vi "CMD_AUTOFOCUS.vi"(6 "Gantry in":refnum<class "Gantry.lvclass">, 8 "error in (no error)":errorcluster, 10 "Arguments":string[](array[string]), 11 "gScript Interpreter in":refnum<class "gScript Interpreter.lvclass">) -> (0 "error out":errorcluster, 3 "gScript Interpreter out":refnum<class "gScript Interpreter.lvclass">, 4 "Gantry out":refnum<class "Gantry.lvclass">)   [LabVIEW 2017, in "gScript Interpreter.lvclass"]
uses:
  gScript Interpreter.lvclass
  Shared Components/Gantry Class/Gantry.lvclass
  Shared Components/Vec3d Class/Vec3d.lvclass
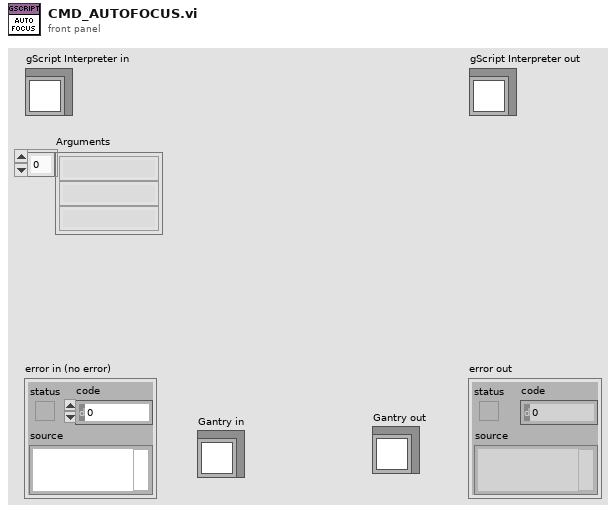
[diagram p1: front panel]
types:
  T1 = typedef "Memory Cell.ctl" = cluster{"type":T2, "x":dbl, "y":dbl, "z":dbl, "w":dbl}
  T2 = typedef "Memory Cell Type Enum.ctl" = enum16{"integer", "float", "vector", "rotation"}
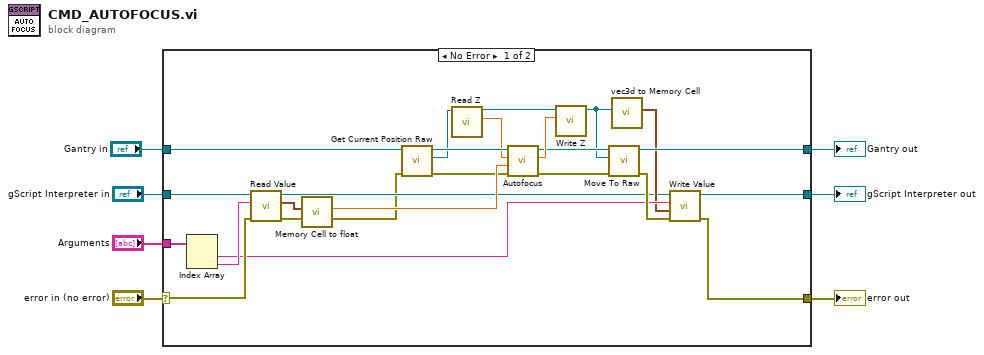
[diagram p0: block diagram]
diagram:
  n1 = case shown="No Error" "error in (no error)" {
    selector: "error in (no error)" -> [w25 w34]
    tunnel: [w27 w34] -> w6
    tunnel: [w29 w33] -> w4
    tunnel: "gScript Interpreter in" -> [w30 w33]
    tunnel: "Arguments" -> [w31 _]
    tunnel: "Gantry in" -> [w26 w32]
    tunnel: [w28 w32] -> w1
    frame No Error {
      n2 = Index Array(array=w31) -> (element #1=w12:string, element #2=w24:string)  [unwired: 2 in]
      n3 = call-dynamic "Read Value.vi"("error in (no error)"=w25, "String in"=w24, "gScript Interpreter in"=w30) -> ("error out"=w8:errorcluster, "Memory Cell"=w22:T1, "gScript Interpreter out"=w9:refnum<class "gScript Interpreter.lvclass">)  [unwired: 6 in]
      n4 = call "Memory Cell to float.vi"("Memory Cell"=w22) -> ("float out"=w23:dbl)  [unwired: 10 in]
      n5 = call-dynamic "Get Current Position Raw.vi"("error in"=w8, "Gantry in"=w26) -> ("error out"=w19:errorcluster, "Vec3d Class out"=w20:refnum<class "Vec3d.lvclass">, "Gantry out"=w21:refnum<class "Gantry.lvclass">)  [unwired: 7 in]
      n6 = call-dynamic "Read Z.vi"("Vec3d Class in"=w20) -> ("Z"=w10:dbl, "Vec3d Class out"=w17:refnum<class "Vec3d.lvclass">)  [unwired: 8 in, 1 out]
      n7 = call "Autofocus.vi"("error in (no error)"=w19, "Range"=w23, "Start Z"=w10, "Gantry in"=w21) -> ("error out"=w15:errorcluster, "focus height"=w18:dbl, "Gantry out"=w16:refnum<class "Gantry.lvclass">)  [unwired: 5 in]
      n8 = call-dynamic "Write Z.vi"("Z"=w18, "Vec3d Class in"=w17) -> ("Vec3d Class out"=w14:refnum<class "Vec3d.lvclass">)  [unwired: 8 in, 1 out]
      n9 = call-dynamic "Move To Raw.vi"("error in"=w15, "Destination"=w14, "Gantry in"=w16) -> ("error out"=w13:errorcluster, "Gantry out"=w28:refnum<class "Gantry.lvclass">)  [unwired: 7 in]
      n10 = call "vec3d to Memory Cell.vi"("Vec3d in"=w14) -> ("Memory Cell"=w11:T1)  [unwired: 10 in]
      n11 = call-dynamic "Write Value.vi"("error in (no error)"=w13, "Value"=w11, "Address"=w12, "gScript Interpreter in"=w9) -> ("error out"=w27:errorcluster, "gScript Interpreter out"=w29:refnum<class "gScript Interpreter.lvclass">)  [unwired: 6 in]
    }
    frame Error {
    }
  }
  "error out" <- w6
  "gScript Interpreter out" <- w4
  "Gantry out" <- w1
